vi "TeleopStateMachine.vi"(0 "QuickTurn":bool, 2 "Camera Toggle":bool, 4 "Intake Speed":dbl, 5 "PincherToggle":bool, 6 "Climber Speed":dbl, 7 "ArmToggle":bool, 8 "GearAim":bool, 9 "PegAim":bool, 10 "Wheel":dbl, 11 "Throttle":dbl) -> (3 "Tele States":T1)   [LabVIEW 2016]
uses:
  TeleStates.ctl
  Robot Global Data.vi
  <vilib>/Rock Robotics/Network Tables/NT Write String.vi
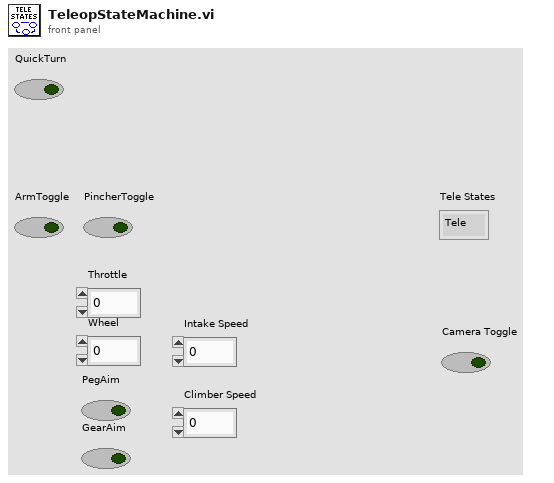
[diagram p1: front panel]
types:
  T1 = typedef "TeleStates.ctl" = enum16{"Tele", "PegAim", "GearAim", "PegForward", "GearForward", "Place", "PegForwardTime", "WaitOnRelease"}
  T2 = cluster{"Target?":bool, "Angle":dbl, "Distance":dbl, "NewAngle":dbl}
  T3 = cluster{"Lower X":dbl, "Lower Y":dbl, "Upper X":dbl, "Upper Y":dbl}
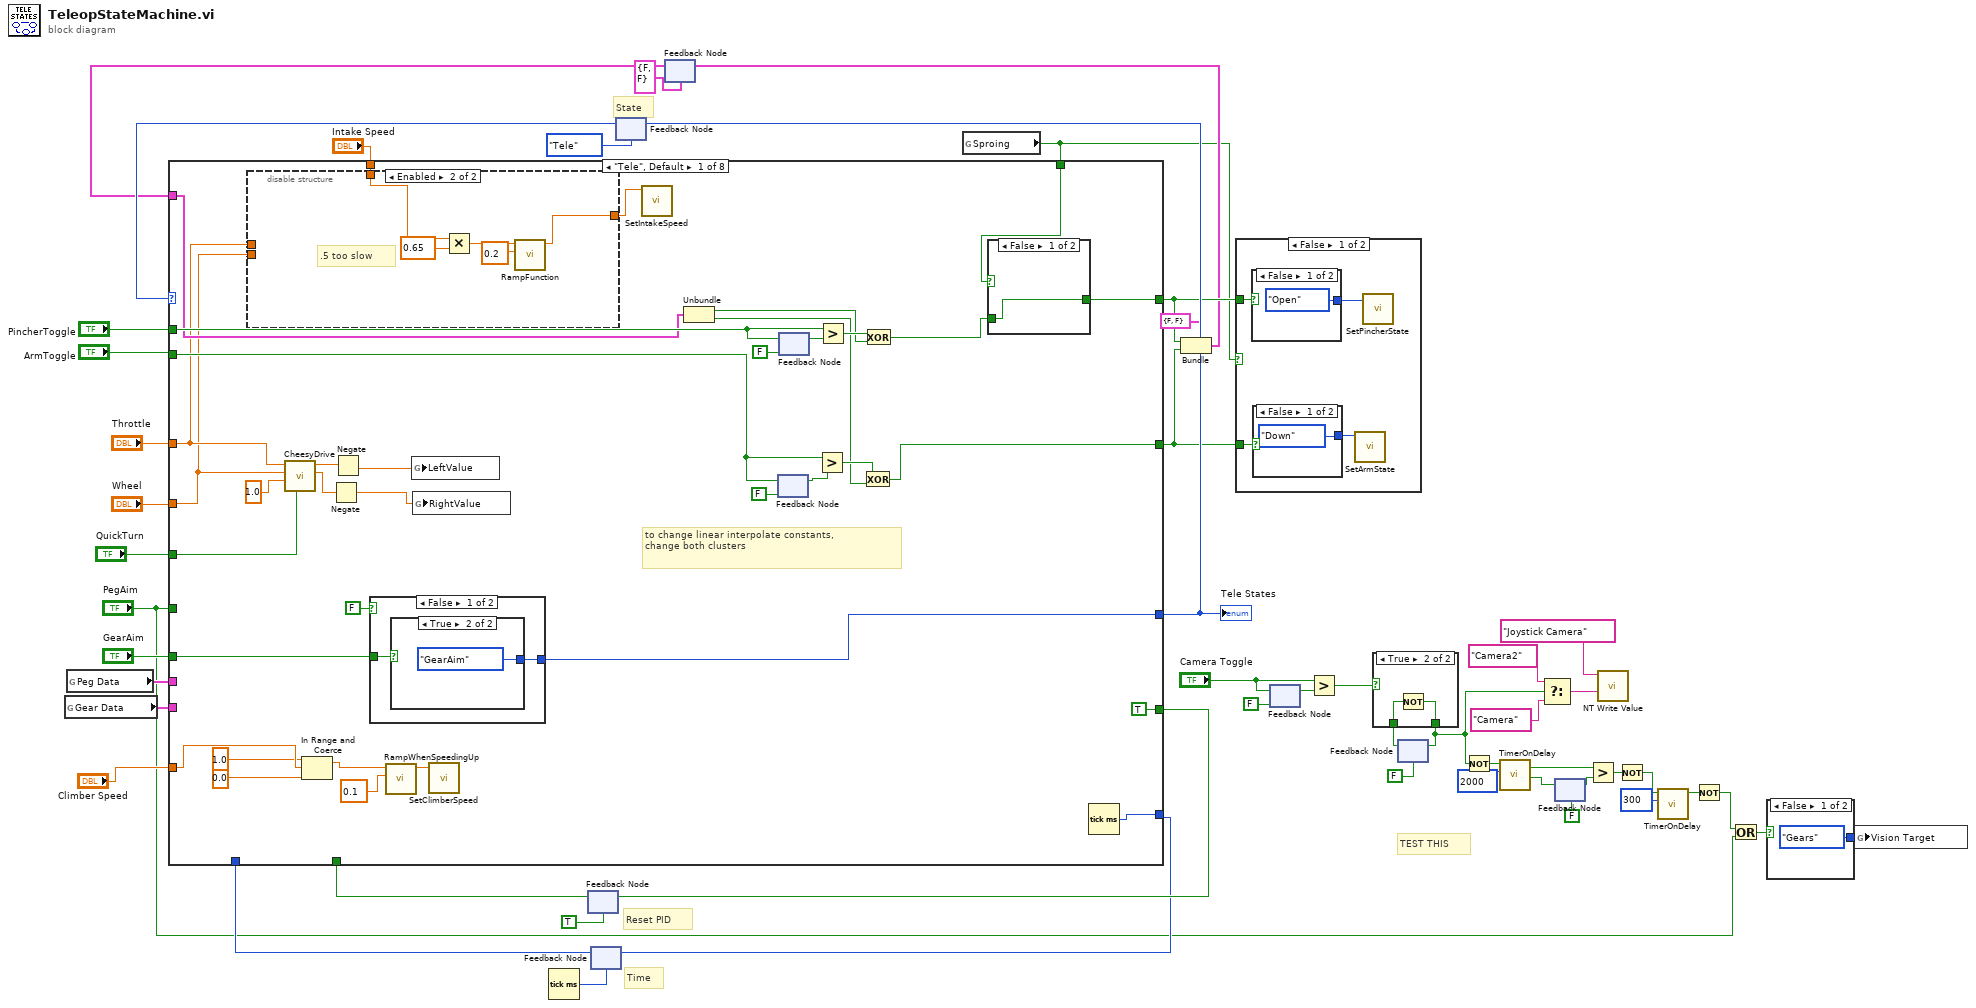
[diagram p0: block diagram]
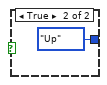
[diagram p2: hidden frame]
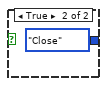
[diagram p3: hidden frame]
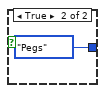
[diagram p5: hidden frame]
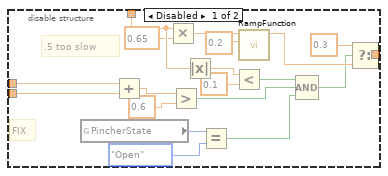
[diagram p7: hidden frame]
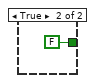
[diagram p8: hidden frame]
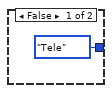
[diagram p9: hidden frame]
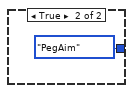
[diagram p10: hidden frame]
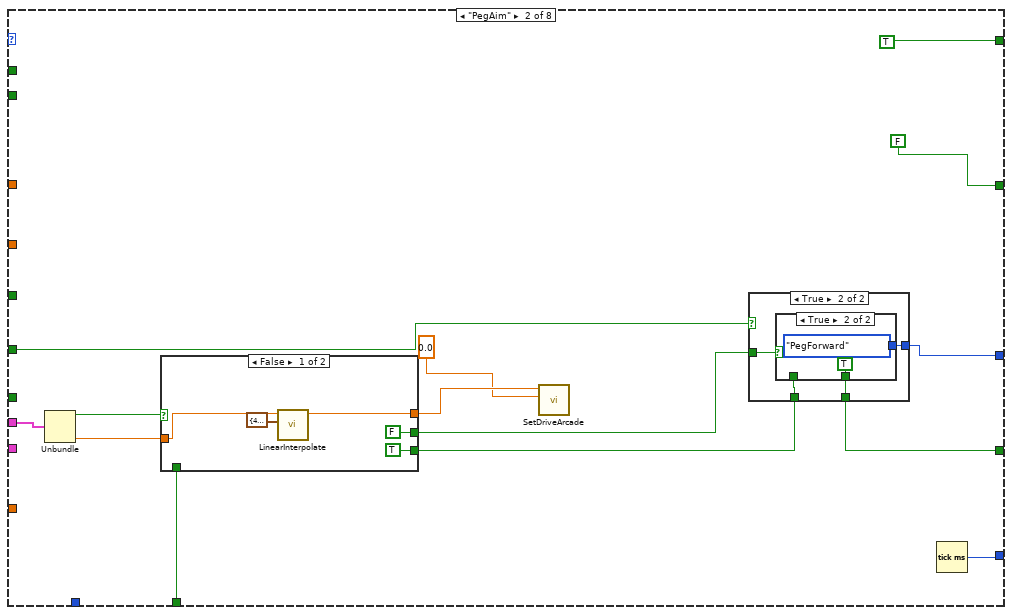
[diagram p11: hidden frame]
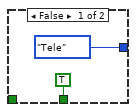
[diagram p12: hidden frame]
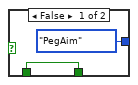
[diagram p13: hidden frame]
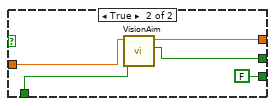
[diagram p14: hidden frame]
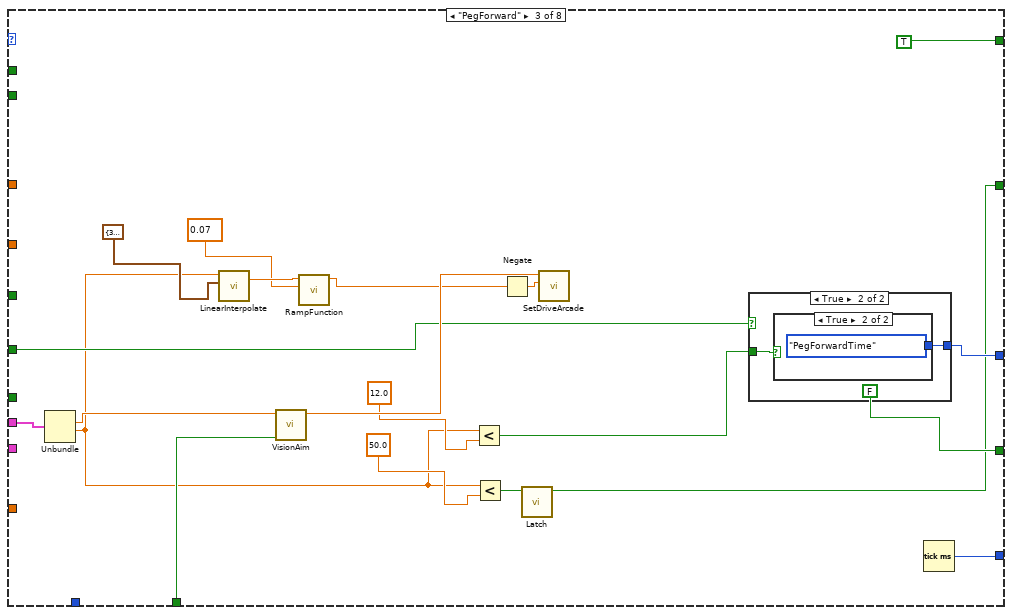
[diagram p15: hidden frame]
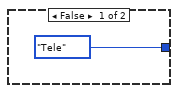
[diagram p16: hidden frame]
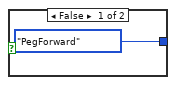
[diagram p17: hidden frame]
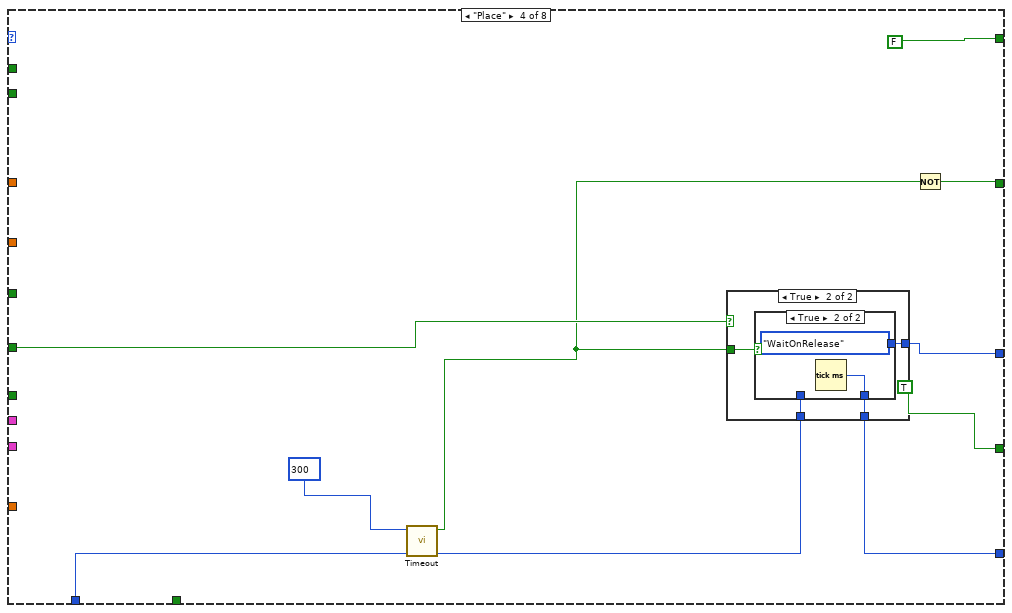
[diagram p18: hidden frame]
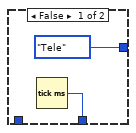
[diagram p19: hidden frame]
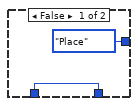
[diagram p20: hidden frame]
diagram:
  # "TEST THIS"
  # "Reset PID"
  # "State"
  # "Time"
  n1 = global read "Robot Global Data.vi" "Gear Data"() -> (w43:T2)
  n2 = global read "Robot Global Data.vi" "Peg Data"() -> (w44:T2)
  n3 = Tick Count (ms)() -> (millisecond timer value=w48:u32)
  n4 = feedback #1(TRUE) -> (w42:bool)
  n5 = feedback #2(w48) -> (w41:u32)
  n6 = feedback #3(TeleStates."Tele" ("Tele States")) -> (w49:T1)
  n7 = feedback #4(cluster{"Pincher":bool, "Arm":bool} {"Pincher"=FALSE, "Arm"=FALSE}) -> (w32:cluster{"Pincher":bool, "Arm":bool})
  n8 = global read "Robot Global Data.vi" "Sproing"() -> (w2:bool)
  n9 = case shown="\"Tele\", Default" w49 {
    tunnel: "PegAim" -> [_ w127 w168 w185 w218 _ _ _]
    tunnel: "GearAim" -> [w86 _ _ _ _ w240 w286 _]
    tunnel: [w85 w126 w167 w186 w219 w244 w296 w315] -> w45
    tunnel: w44 -> [_ w131 w171 _ _ _ _ _]
    tunnel: w43 -> [_ _ _ _ _ w241 w287 _]
    tunnel: w42 -> [_ w124 w166 _ _ w242 w295 _]
    tunnel: w41 -> [_ _ _ w183 w216 _ _ _]
    tunnel: [TRUE w120 FALSE TRUE TRUE w245 w297 TRUE] -> w40
    tunnel: [w84 w123 w159 w180 w213 w239 w285 w320] -> w39
    tunnel: "ArmToggle" -> [w79 _ _ _ _ _ _ w318]
    tunnel: "PincherToggle" -> [w75 _ _ _ _ _ _ w319]
    tunnel: [w59 TRUE TRUE FALSE w197 FALSE w283 w323] -> w36
    tunnel: [w74 FALSE w152 w178 TRUE FALSE FALSE w322] -> w35
    tunnel: w32 -> [w73 _ _ _ _ _ _ w324]
    tunnel: "Intake Speed" -> [w63 _ _ _ _ _ _ _]
    tunnel: "Throttle" -> [w58 _ _ _ _ w235 _ _]
    tunnel: "Wheel" -> [w57 _ _ _ _ w236 _ _]
    tunnel: "Climber Speed" -> [w67 _ _ _ _ _ _ _]
    tunnel: w2 -> [w61 _ _ _ _ _ _ _]
    tunnel: "QuickTurn" -> [w52 _ _ _ _ _ _ _]
    frame "Tele", Default {
      # "to change linear interpolate constants,\nchange both clusters"
      n10 = disable-structure shown="Enabled" {
        disable-tunnel: [w94 w106] -> w68
        disable-tunnel: w63 -> [w90 w107]
        disable-tunnel: w58 -> [w88 _]
        disable-tunnel: w57 -> [w87 _]
        frame Disabled {
          # "FIX"
          # ".5 too slow"
          n11 = global read "Robot Global Data.vi" "PincherState"() -> (w97:enum16{"Open", "Close"})
          n12 = Add(x=w88, y=w87) -> (x+y=w100:dbl)
          n13 = Multiply(x=w90, y=0.65) -> (x*y=w104:dbl)
          n14 = Greater?(x=w100, y=0.6) -> (0:w98:bool)
          n15 = Absolute Value(x=w90) -> (abs(x)=w103:dbl)
          n16 = Equal?(x=w97, y=enum16{"Open", "Close"}."Open") -> (x = y?=w95:bool)
          n17 = Less?(x=w103, y=0.1) -> (x < y?=w101:bool)
          n18 = call "RampFunction.vi"("Max Rate"=0.2, "Input"=w104) -> ("Output"=w93:dbl)  [unwired: 9 in]
          n19 = Compound Arithmetic op=AND(w101, w98, w95) -> (w91:bool)
          n20 = Select(t=0.3, s=w91, f=w93) -> (s? t:f=w94:dbl)
        }
        frame Enabled {
          # ".5 too slow"
          n21 = Multiply(x=w107, y=0.65) -> (x*y=w109:dbl)
          n22 = call "RampFunction.vi"("Max Rate"=0.2, "Input"=w109) -> ("Output"=w106:dbl)  [unwired: 9 in]
        }
      }
      n23 = call "CheesyDrive.vi"("Quickturn"=w52, "Sensitivty"=1.0 ("Wheel"), "Wheel"=w57, "Throttle"=w58) -> ("Right PWM"=w55:dbl, "Left PWM"=w56:dbl)  [unwired: 6 in]
      n24 = In Range and Coerce(upper limit=1.0, x=w67, lower limit=0.0) -> (coerced(x)=w64:dbl)  [unwired: 1 out]
      n25 = Negate(x=w55) -> (-x=w53:dbl)
      n26 = Negate(x=w56) -> (-x=w54:dbl)
      n27 = case shown="False" FALSE {
        tunnel: [w113 TeleStates."PegAim" ("Tele States")] -> w85
        tunnel: w86 -> [w114 _]
        frame False {
          n28 = case shown="True" w114 {
            tunnel: [TeleStates."Tele" ("Tele States") TeleStates."GearAim" ("Tele States")] -> w113
            frame False {
            }
            frame True {
            }
          }
        }
        frame True {
        }
      }
      n29 = call "RampWhenSpeedingUp.vi"("Ramp"=0.1, "Input"=w64) -> ("Output"=w69:dbl)  [unwired: 9 in]
      n30 = global write "Robot Global Data.vi" "LeftValue"(w54) -> ()
      n31 = global write "Robot Global Data.vi" "RightValue"(w53) -> ()
      n32 = call "SetClimberSpeed.vi"("ClimberSpeed"=w69) -> ()  [unwired: 10 in, 1 out]
      n33 = call "SetIntakeSpeed.vi"("Speed"=w68) -> ()  [unwired: 10 in, 1 out]
      n34 = Unbundle(w73) -> ("Pincher"=w72:bool, "Arm"=w71:bool)
      n35 = feedback #5(FALSE) -> (w81:bool)
      n36 = feedback-in #5(w79) -> ()
      n37 = feedback #6(FALSE) -> (w77:bool)
      n38 = feedback-in #6(w75) -> ()
      n39 = Greater?(x=w79, y=w81) -> (0:w80:bool)
      n40 = Greater?(x=w75, y=w77) -> (0:w76:bool)
      n41 = Exclusive Or(1:w71, 2:w80) -> (0:w74:bool)
      n42 = Exclusive Or(1:w72, 2:w76) -> (0:w60:bool)
      n43 = case shown="False" w61 {
        tunnel: w60 -> [w111 _]
        tunnel: [w111 FALSE] -> w59
        frame False {
        }
        frame True {
        }
      }
      n44 = Tick Count (ms)() -> (millisecond timer value=w84:u32)
    }
    frame "PegAim" {
      n45 = Unbundle(w131) -> ("Target?"=w130:bool, "NewAngle"=w122:dbl)  [unwired: 2 out]
      n46 = case shown="False" w130 {
        tunnel: [w146 w150] -> w129
        tunnel: w122 -> [w145 w151]
        tunnel: [FALSE w148] -> w125
        tunnel: [TRUE FALSE] -> w121
        tunnel: w124 -> [_ w147]
        frame False {
          n47 = call "LinearInterpolate.vi"("Config"=T3 {"Lower X"=45.0, "Lower Y"=0.5, "Upper X"=110.0, "Upper Y"=0.85}, "Value"=w145) -> ("Output"=w146:dbl)  [unwired: 9 in]
        }
        frame True {
          n48 = call "VisionAim.vi"("Reset PID"=w147, "Angle"=w151) -> ("In Range"=w148:bool, "Turn"=w150:dbl)  [unwired: 8 in]
        }
      }
      n49 = call "SetDriveArcade.vi"("Forward"=0.0, "Turn"=w129) -> ()  [unwired: 9 in, 1 out]
      n50 = case shown="True" w127 {
        tunnel: [TeleStates."Tele" ("Tele States") w137] -> w126
        tunnel: w125 -> [_ w136]
        tunnel: w121 -> [_ w135]
        tunnel: [TRUE w134] -> w120
        frame False {
        }
        frame True {
          n51 = case shown="True" w136 {
            tunnel: [TeleStates."PegAim" ("Tele States") TeleStates."PegForward" ("Tele States")] -> w137
            tunnel: w135 -> [w138 _]
            tunnel: [w138 TRUE] -> w134
            frame False {
            }
            frame True {
            }
          }
        }
      }
      n52 = Tick Count (ms)() -> (millisecond timer value=w123:u32)
    }
    frame "PegForward" {
      n53 = Unbundle(w171) -> ("Angle"=w158:dbl, "Distance"=w156:dbl)  [unwired: 2 out]
      n54 = call "LinearInterpolate.vi"("Config"=T3 {"Lower X"=30.0, "Lower Y"=0.5, "Upper X"=50.0, "Upper Y"=0.7}, "Value"=w156) -> ("Output"=w162:dbl)  [unwired: 9 in]
      n55 = call "VisionAim.vi"("Reset PID"=w166, "Angle"=w158) -> ("Turn"=w170:dbl)  [unwired: 8 in, 1 out]
      n56 = call "RampFunction.vi"("Max Rate"=0.07, "Input"=w162) -> ("Output"=w160:dbl)  [unwired: 9 in]
      n57 = Less?(x=w156, y=12.0) -> (x < y?=w155:bool)
      n58 = Less?(x=w156, y=50.0) -> (x < y?=w153:bool)
      n59 = Negate(x=w160) -> (-x=w163:dbl)
      n60 = call "Latch.vi"("Input"=w153) -> ("Output"=w152:bool)  [unwired: 10 in]
      n61 = call "SetDriveArcade.vi"("Forward"=w163, "Turn"=w170) -> ()  [unwired: 9 in, 1 out]
      n62 = case shown="True" w168 {
        tunnel: [TeleStates."Tele" ("Tele States") w174] -> w167
        tunnel: w155 -> [_ w173]
        frame False {
        }
        frame True {
          n63 = case shown="True" w173 {
            tunnel: [TeleStates."PegForward" ("Tele States") TeleStates."PegForwardTime" ("Tele States")] -> w174
            frame False {
            }
            frame True {
            }
          }
        }
      }
      n64 = Tick Count (ms)() -> (millisecond timer value=w159:u32)
    }
    frame "Place" {
      n65 = call "Timeout.vi"("Start Time In"=w183, "Time Limit (ms)"=u32 300 ("Time Limit")) -> ("Start Time Out"=w181:u32, "Timeout"=w177:bool)  [unwired: 8 in]
      n66 = case shown="True" w185 {
        tunnel: [TeleStates."Tele" ("Tele States") w192] -> w186
        tunnel: w177 -> [_ w191]
        tunnel: w181 -> [_ w190]
        tunnel: [w187 w189] -> w180
        frame False {
          n67 = Tick Count (ms)() -> (millisecond timer value=w187:u32)
        }
        frame True {
          n68 = case shown="True" w191 {
            tunnel: [TeleStates."Place" ("Tele States") TeleStates."WaitOnRelease" ("Tele States")] -> w192
            tunnel: w190 -> [w193 _]
            tunnel: [w193 w196] -> w189
            frame False {
            }
            frame True {
              n69 = Tick Count (ms)() -> (millisecond timer value=w196:u32)
            }
          }
        }
      }
      n70 = Not(x=w177) -> (.not. x?=w178:bool)
    }
    frame "PegForwardTime" {
      w199 = 0.55 ("Forward")
      n71 = Tick Count (ms)() -> (millisecond timer value=w208:u32)
      n72 = Negate(x=w199) -> (-x=w200:dbl)
      n73 = feedback #7(w208) -> (w206:u32)
      n74 = call "Timeout.vi"("Start Time In"=w206, "Time Limit (ms)"=u32 300 ("Time Limit")) -> ("Start Time Out"=w209:u32, "Timeout"=w210:bool)  [unwired: 8 in]
      n75 = feedback #8(FALSE) -> (w204:bool)
      n76 = case shown="True" w210 {
        tunnel: w204 -> [w221 w224]
        tunnel: [w221 w223] -> w205
        tunnel: w209 -> [w220 _]
        tunnel: [w220 w222] -> w207
        frame False {
        }
        frame True {
          n77 = Not(x=w224) -> (.not. x?=w223:bool)
          n78 = Tick Count (ms)() -> (millisecond timer value=w222:u32)
        }
      }
      n79 = feedback-in #7(w207) -> ()
      n80 = feedback-in #8(w205) -> ()
      n81 = call "Timeout.vi"("Start Time In"=w216, "Time Limit (ms)"=u32 1700 ("Time Limit")) -> ("Start Time Out"=w214:u32, "Timeout"=w198:bool)  [unwired: 8 in]
      n82 = Select(t=w199, s=w205, f=w200) -> (s? t:f=w211:dbl)
      n83 = call "SetDriveArcade.vi"("Forward"=-0.55, "Turn"=w211) -> ()  [unwired: 9 in, 1 out]
      n84 = case shown="True" w218 {
        tunnel: [TeleStates."Tele" ("Tele States") w230] -> w219
        tunnel: w198 -> [_ w229]
        tunnel: w214 -> [_ w228]
        tunnel: [w225 w227] -> w213
        frame False {
          n85 = Tick Count (ms)() -> (millisecond timer value=w225:u32)
        }
        frame True {
          n86 = case shown="True" w229 {
            tunnel: [TeleStates."PegForwardTime" ("Tele States") TeleStates."Place" ("Tele States")] -> w230
            tunnel: w228 -> [w232 _]
            tunnel: [w232 w233] -> w227
            frame False {
            }
            frame True {
              n87 = Tick Count (ms)() -> (millisecond timer value=w233:u32)
            }
          }
        }
      }
      n88 = Not(x=w198) -> (.not. x?=w197:bool)
    }
    frame "GearAim" {
      n89 = Unbundle(w241) -> ("Target?"=w247:bool, "Angle"=w246:dbl)  [unwired: 2 out]
      n90 = case shown="True" w247 {
        tunnel: w246 -> [_ w282]
        tunnel: [FALSE w280] -> w243
        tunnel: [TRUE FALSE] -> w245
        tunnel: w242 -> [_ w279]
        tunnel: w236 -> [w255 _]
        tunnel: w235 -> [w254 _]
        frame False {
          w253 = T3 {"Lower X"=0.07, "Lower Y"=0.35, "Upper X"=1.0, "Upper Y"=1.0} ("Config")
          w266 = 0.2 ("Max Rate")
          # "Driver turns robot"
          n91 = Absolute Value(x=w255) -> (abs(x)=w258:dbl)
          n92 = Absolute Value(x=w254) -> (abs(x)=w263:dbl)
          n93 = Less?(x=w258, y=0.07) -> (x < y?=w257:bool)
          n94 = Less?(x=w263, y=0.07) -> (x < y?=w261:bool)
          n95 = case shown="False" w261 {
            tunnel: w254 -> [w275 _]
            tunnel: w253 -> [w274 _]
            tunnel: [w273 0.0 ("Output")] -> w260
            frame False {
              n96 = call "LinearInterpolate.vi"("Config"=w274, "Value"=w275) -> ("Output"=w273:dbl)  [unwired: 9 in]
            }
            frame True {
            }
          }
          n97 = case shown="False" w257 {
            tunnel: w255 -> [w271 _]
            tunnel: [w270 0.0 ("Output")] -> w256
            tunnel: w253 -> [w269 _]
            frame False {
              n98 = call "LinearInterpolate.vi"("Config"=w269, "Value"=w271) -> ("Output"=w270:dbl)  [unwired: 9 in]
            }
            frame True {
            }
          }
          n99 = call "RampWhenSpeedingUp.vi"("Ramp"=w266, "Input"=w260) -> ("Output"=w265:dbl)  [unwired: 9 in]
          n100 = call "RampWhenSpeedingUp.vi"("Ramp"=w266, "Input"=w256) -> ("Output"=w264:dbl)  [unwired: 9 in]
          n101 = call "SetDriveTank.vi"("Right"=w264, "Left"=w265) -> ()  [unwired: 9 in, 1 out]
        }
        frame True {
          n102 = call "VisionAim.vi"("Reset PID"=w279, "Angle"=w282) -> ("In Range"=w280:bool, "Turn"=w277:dbl)  [unwired: 8 in]
          n103 = call "SetDriveArcade.vi"("Forward"=0.0, "Turn"=w277) -> ()  [unwired: 9 in, 1 out]
        }
      }
      n104 = case shown="True" w240 {
        tunnel: [TeleStates."Tele" ("Tele States") w250] -> w244
        tunnel: w243 -> [_ w249]
        frame False {
        }
        frame True {
          n105 = case shown="True" w249 {
            tunnel: [TeleStates."GearAim" ("Tele States") TeleStates."GearForward" ("Tele States")] -> w250
            frame False {
            }
            frame True {
            }
          }
        }
      }
      n106 = Tick Count (ms)() -> (millisecond timer value=w239:u32)
    }
    frame "GearForward" {
      n107 = Unbundle(w287) -> ("Target?"=w300:bool, "Angle"=w298:dbl, "Distance"=w292:dbl)  [unwired: 1 out]
      n108 = case shown="False" w300 {
        tunnel: [w309 w312] -> w299
        tunnel: w298 -> [w308 w313]
        tunnel: [TRUE FALSE] -> w297
        tunnel: w295 -> [_ w310]
        frame False {
          n109 = call "LinearInterpolate.vi"("Config"=T3 {"Lower X"=45.0, "Lower Y"=0.5, "Upper X"=110.0, "Upper Y"=0.85}, "Value"=w308) -> ("Output"=w309:dbl)  [unwired: 9 in]
        }
        frame True {
          n110 = call "VisionAim.vi"("Reset PID"=w310, "Angle"=w313) -> ("Turn"=w312:dbl)  [unwired: 8 in, 1 out]
        }
      }
      n111 = call "LinearInterpolate.vi"("Config"=T3 {"Lower X"=0.0, "Lower Y"=0.5, "Upper X"=60.0, "Upper Y"=0.65}, "Value"=w292) -> ("Output"=w290:dbl)  [unwired: 9 in]
      n112 = call "RampFunction.vi"("Max Rate"=0.07, "Input"=w290) -> ("Output"=w288:dbl)  [unwired: 9 in]
      n113 = Less?(x=w292, y=-5.0) -> (x < y?=w283:bool)
      n114 = Negate(x=w288) -> (-x=w291:dbl)
      n115 = call "SetDriveArcade.vi"("Forward"=w291, "Turn"=w299) -> ()  [unwired: 9 in, 1 out]
      n116 = case shown="True" w286 {
        tunnel: [TeleStates."Tele" ("Tele States") w303] -> w296
        tunnel: w283 -> [_ w302]
        frame False {
        }
        frame True {
          n117 = case shown="True" w302 {
            tunnel: [TeleStates."GearForward" ("Tele States") TeleStates."WaitOnRelease" ("Tele States")] -> w303
            frame False {
            }
            frame True {
            }
          }
        }
      }
      n118 = Tick Count (ms)() -> (millisecond timer value=w285:u32)
    }
    frame "WaitOnRelease" {
      n119 = Not(x=w319) -> (.not. x?=w316:bool)
      n120 = Not(x=w318) -> (.not. x?=w317:bool)
      n121 = Unbundle(w324) -> ("Pincher"=w323:bool, "Arm"=w322:bool)
      n122 = And(x=w316, y=w317) -> (x .and. y?=w314:bool)
      n123 = case shown="False" w314 {
        tunnel: [TeleStates."WaitOnRelease" ("Tele States") TeleStates."Tele" ("Tele States")] -> w315
        frame False {
        }
        frame True {
        }
      }
      n124 = Tick Count (ms)() -> (millisecond timer value=w320:u32)
    }
  }
  "Tele States" <- w45
  n125 = feedback-in #1(w40) -> ()
  n126 = feedback-in #2(w39) -> ()
  n127 = feedback-in #3(w45) -> ()
  n128 = Bundle(cluster=cluster{"Pincher":bool, "Arm":bool} {"Pincher"=FALSE, "Arm"=FALSE}, "Pincher"=w36, "Arm"=w35) -> (w33:cluster{"Pincher":bool, "Arm":bool})
  n129 = feedback-in #4(w33) -> ()
  n130 = case shown="False" w2 {
    tunnel: w36 -> [w328 _]
    tunnel: w35 -> [w327 _]
    frame False {
      n131 = case shown="False" w328 {
        tunnel: [enum16{"Open", "Close"}."Open" ("PincherState") enum16{"Open", "Close"}."Close" ("PincherState")] -> w330
        frame False {
        }
        frame True {
        }
      }
      n132 = case shown="False" w327 {
        tunnel: [enum16{"Up", "Down"}."Down" ("ArmState") enum16{"Up", "Down"}."Up" ("ArmState")] -> w329
        frame False {
        }
        frame True {
        }
      }
      n133 = call "SetArmState.vi"("ArmState"=w329) -> ()  [unwired: 10 in, 1 out]
      n134 = call "SetPincherState.vi"("PincherState"=w330) -> ()  [unwired: 10 in, 1 out]
    }
    frame True {
    }
  }
  n135 = feedback #9(FALSE) -> (w18:bool)
  n136 = feedback-in #9("Camera Toggle") -> ()
  n137 = Greater?(x="Camera Toggle", y=w18) -> (0:w19:bool)
  n138 = feedback #10(FALSE ("Front Camera")) -> (w21:bool)
  n139 = case shown="True" w19 {
    tunnel: w21 -> [w335 w337]
    tunnel: [w335 w336] -> w13
    frame False {
    }
    frame True {
      n140 = Not(x=w337) -> (.not. x?=w336:bool)
    }
  }
  n141 = feedback-in #10(w13) -> ()
  n142 = Not(x=w13) -> (.not. x?=w12:bool)
  n143 = call "TimerOnDelay.vi"("Time Limit"=u32 2000, "Input"=w12) -> ("Output"=w11:bool)  [unwired: 9 in]
  n144 = Select(t="Camera2", s=w13, f="Camera") -> (s? t:f=w25:string)
  n145 = feedback #11(FALSE) -> (w14:bool)
  n146 = feedback-in #11(w11) -> ()
  n147 = Greater?(x=w11, y=w14) -> (0:w7:bool)
  n148 = call-poly <vilib>:"NT Write Value.vi"("String"=w25, "Name"="Joystick Camera") -> ()  [unwired: 9 in, 1 out]
  n149 = Not(x=w7) -> (.not. x?=w6:bool)
  n150 = call "TimerOnDelay.vi"("Time Limit"=u32 300, "Input"=w6) -> ("Output"=w4:bool)  [unwired: 9 in]
  n151 = Not(x=w4) -> (.not. x?=w3:bool)
  n152 = Or(x=w3, y="PegAim") -> (x .or. y?=w9:bool)
  n153 = case shown="False" w9 {
    tunnel: [enum16{"Pegs", "Gears"}."Gears" ("Vision Target") enum16{"Pegs", "Gears"}."Pegs" ("Vision Target")] -> w16
    frame False {
    }
    frame True {
    }
  }
  n154 = global write "Robot Global Data.vi" "Vision Target"(w16) -> ()
